vi "Initialize.vi"(8 "error in (no error)":errorcluster, 10 "Name":string, 11 "DataShare in":refnum<class "DataShare.lvclass">) -> (0 "error out":errorcluster, 3 "DataShare out":refnum<class "DataShare.lvclass">)   [LabVIEW 2016, in "DataShare.lvclass"]
uses:
  DataShare.lvclass
  DataShare.lvclass/DataShare.ctl
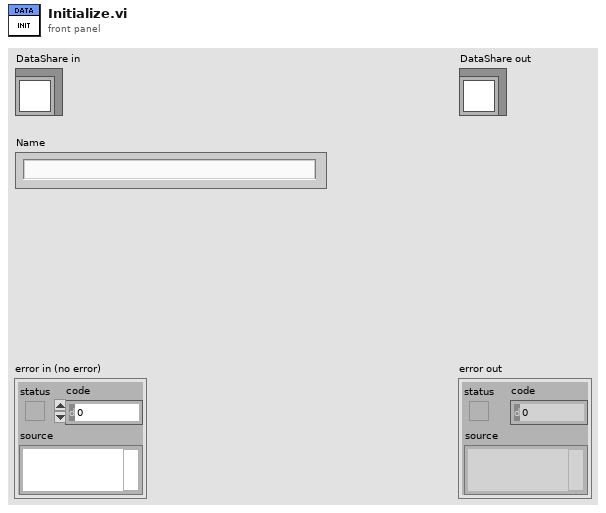
[diagram p1: front panel]
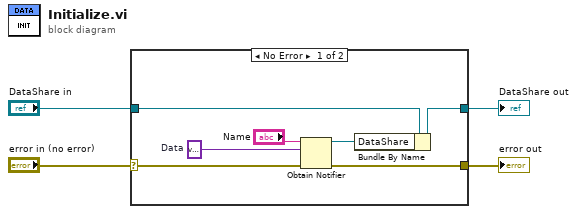
[diagram p0: block diagram]
diagram:
  n1 = case shown="No Error" "error in (no error)" {
    selector: "error in (no error)" -> [w10 w13]
    tunnel: [w9 w13] -> w3
    tunnel: [w7 w12] -> w1
    tunnel: "DataShare in" -> [w8 w12]
    frame No Error {
      w6 = variant  # Data
      n2 = Obtain Notifier(name (unnamed)="Name", notification data type=w6, error in (no error)=w10) -> (notifier out=w5:refnum<notifier>, error out=w9:errorcluster)  [unwired: 1 in, 1 out]
      n3 = Bundle By Name(cluster=w8, "DataShare"=w5) -> (w7:refnum<class "DataShare.lvclass">)
    }
    frame Error {
    }
  }
  "error out" <- w3
  "DataShare out" <- w1
